vi "NotifyIcon - Example 2.vi"() -> ()   [LabVIEW 2018]
uses:
  TypeDefs/NotifyIcon Events.ctl
  TypeDefs/NotifyIcon Event Registration Actions.ctl
  System.Windows.Forms
panel:
  in  "Events to register":T1[](array[typedef])=[enum."BalloonTipClosed"]
  in  "Add to Event Registration":bool
  in  "Checked":bool
  in  "Visible":bool=TRUE
  in  "Context MenuItem":string="submenu\\subitem1"
  in  "Change MenuItem Properties":bool
  in  "New Icon File Path":path=path "C:/Program Files/National Instruments/LabVIEW 2009/applibs/lvapp.ico"
  in  "Change Icon":bool
  in  "Context Menu":string[][](array[string])=[["<submenu2>", "<submenu1>", "<submenu2>"], ["<submenu1>", "subitem1", "subitem1"], ["item1", "subitem2", "subitem2"], ["item2", "", "subitem3"], ["-", "", ""], ["Exit", "", ""]]
  in  "Change Context Menu":bool
  in  "Text":string="Baloon Tip Text"
  in  "Title":string="Balloon Tip"
  in  "Icon (None)":i32(ring)=1 items=["None", "Info", "Warning", "Error"]
  in  "Show Balloon Tip":bool
  in  "stop":bool
  in  "Icon File Path (set to valid path before running)":path=path "C:/Program Files/National Instruments/LabVIEW 2009/applibs/lvapp.ico"
  # "**Warning - if you register a new event, you need to handle the\nevent in the Case Structure found in the NotifyIcon User Event.\n\nIf you do not, you will recieve error 7000"
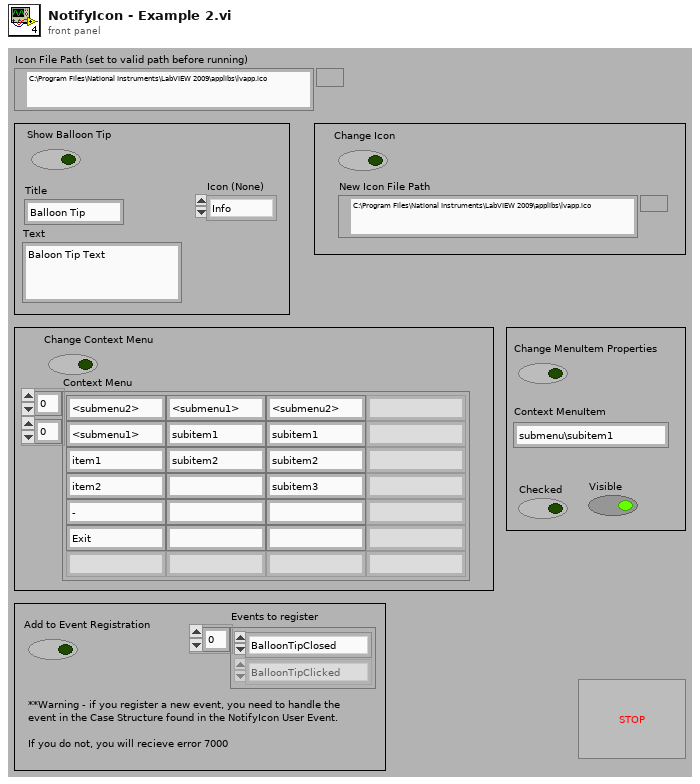
[diagram p1: front panel]
types:
  T1 = typedef "NotifyIcon Events.ctl" = enum16{"BalloonTipClicked", "BalloonTipClosed", "BalloonTipShown", "Click", "Disposed", "DoubleClick", "MouseClick", "MouseDoubleClick", "MouseDown", "MouseMove", "MouseUp", "MenuItemClick", "MenuItemSelect"}
  T2 = typedef "NotifyIcon Event Registration Actions.ctl" = enum16{"Initial Event Registration", "Add to Event Registration", "Destroy Events and Re-register"}
  T3 = typedef "NotifyIcon Event Data.ctl" = cluster{"NotifyIcon Event":T1, "Data String":string}
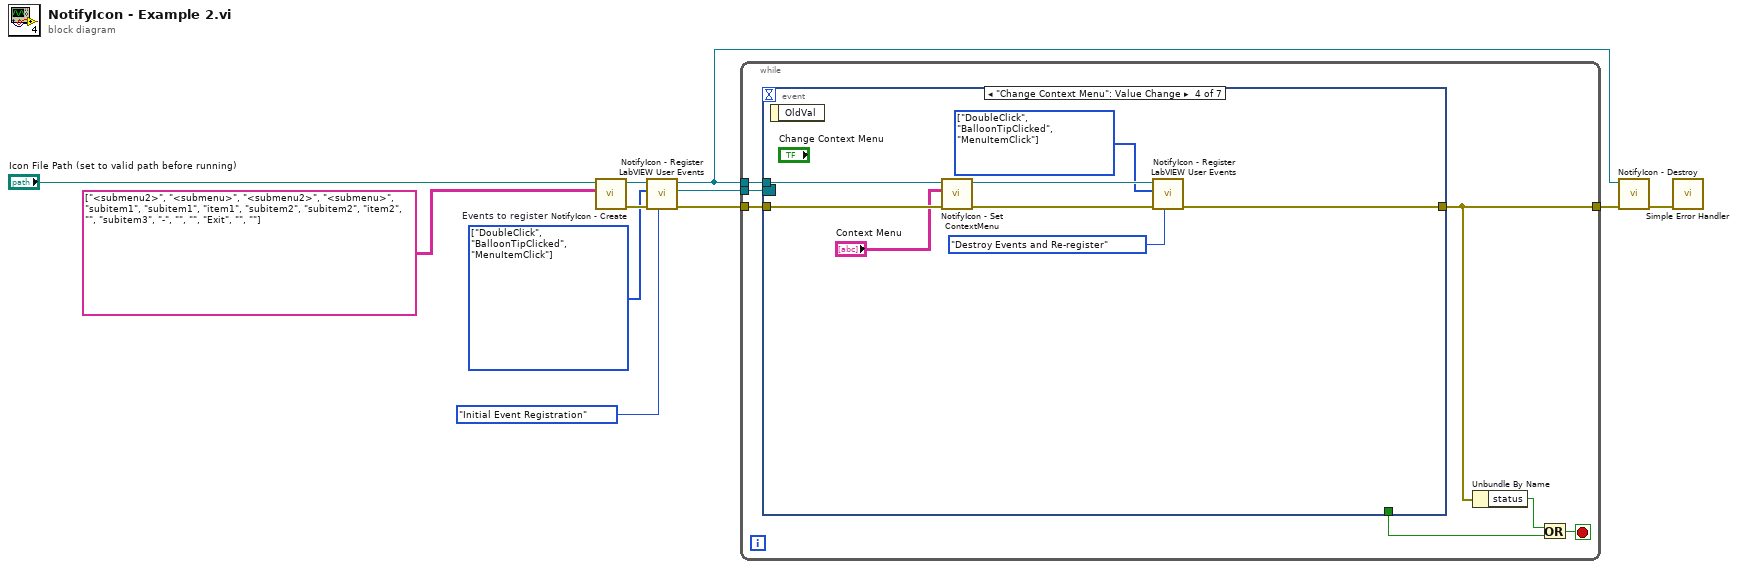
[diagram p0: block diagram]
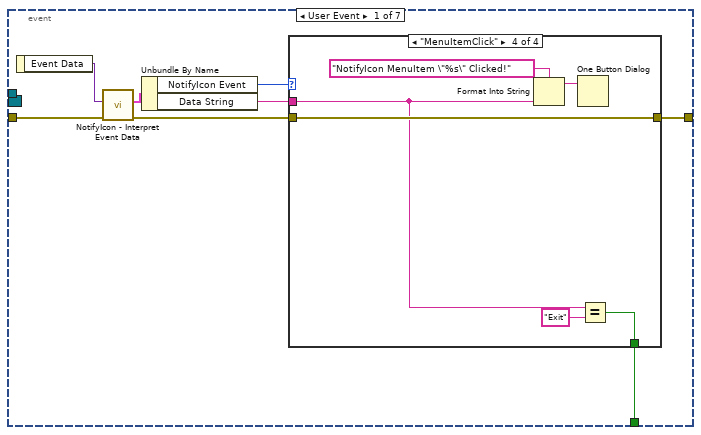
[diagram p2: hidden frame]
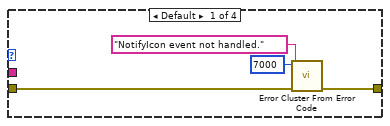
[diagram p3: hidden frame]
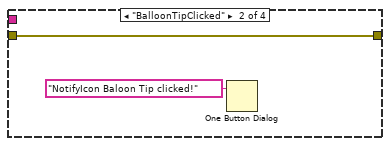
[diagram p4: hidden frame]
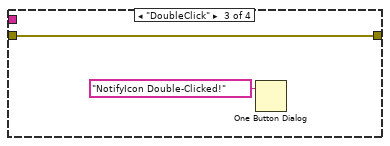
[diagram p5: hidden frame]
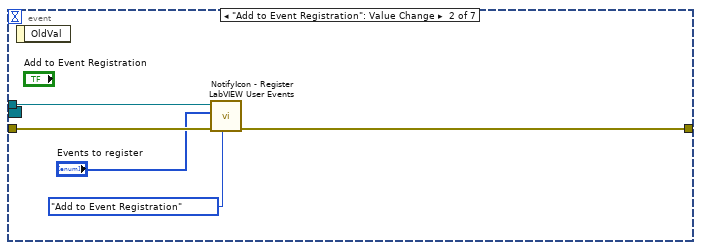
[diagram p6: hidden frame]
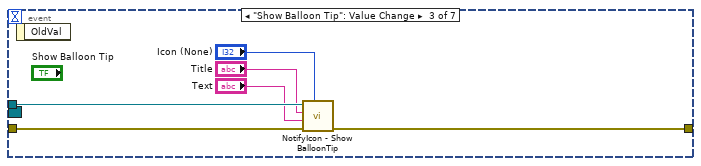
[diagram p7: hidden frame]
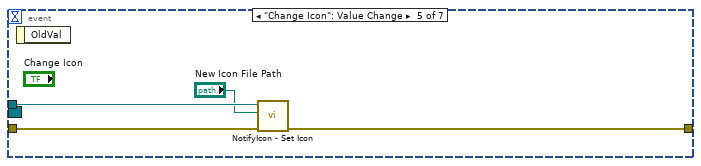
[diagram p8: hidden frame]
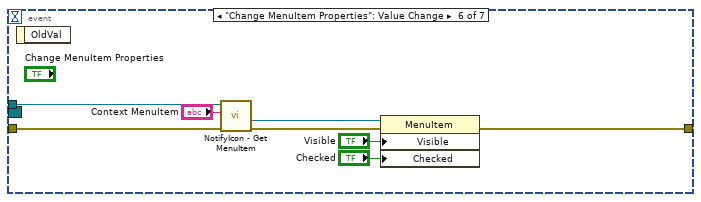
[diagram p9: hidden frame]
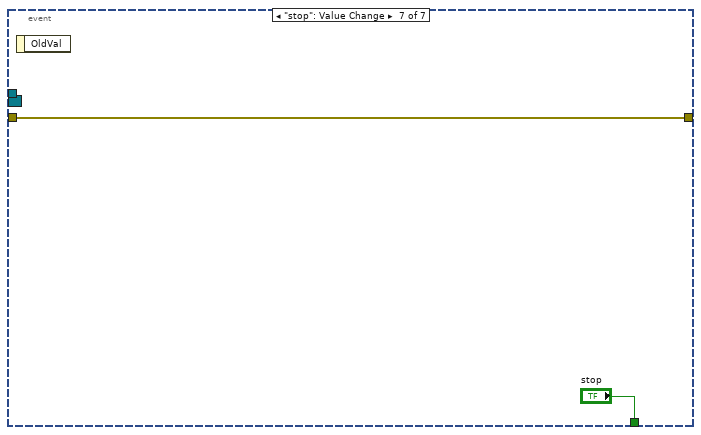
[diagram p10: hidden frame]
diagram:
  w8 = T1[] [enum."DoubleClick", enum."BalloonTipClicked", enum."MenuItemClick"] items=["BalloonTipClicked", "BalloonTipClosed", "BalloonTipShown", "Click", "Disposed", "DoubleClick", "MouseClick", "MouseDoubleClick", "MouseDown", "MouseMove", "MouseUp", "MenuItemClick", "MenuItemSelect"]  # Events to register
  n1 = call "NotifyIcon - Create.vi"("Context Menu (optional)"=string[][] [["<submenu2>", "<submenu>", "<submenu2>"], ["<submenu>", "subitem1", "subitem1"], ["item1", "subitem2", "subitem2"], ["item2", "", "subitem3"], ["-", "", ""], ["Exit", "", ""]], "Icon File Path"="Icon File Path (set to valid path before running)") -> ("error out"=w9:errorcluster, "NotifyIcon reference"=w11:refnum<k24>)  [unwired: 8 in]
  n2 = call "NotifyIcon - Register LabVIEW User Events.vi"("Action"=NotifyIcon_Event_Registration_Actions."Initial Event Registration", "error in"=w9, "Events to register"=w8, "NotifyIcon reference in"=w11) -> ("error out"=w5:errorcluster, "Event Registration Refnum"=w6:refnum<event-registration>, "NotifyIcon reference out"=w2:refnum<k24>)  [unwired: 5 in]
  n3 = while {
    tunnel: w6 -> [w18]
    tunnel: w2 -> [w17]
    tunnel: w5 -> [w16]
    tunnel: [w12] -> w4
    stop <- w13 stop-if-true
    n4 = event shown="[3] \"Change Context Menu\": Value Change" {
      selector: w18 -> [_ _ _ _ _ _ _]
      dyn-events: _ -> [_ _ _ _ _ _ _]
      timeout: _ -> [_ _ _ _ _ _ _]
      tunnel: w17 -> [_ w45 w50 w58 w63 w70 _]
      tunnel: w16 -> [w26 w44 w51 w59 w62 w71 w72]
      tunnel: [w19 _ _ _ _ _ "stop"] -> w15
      tunnel: [w21 w42 w46 w52 w60 w67 w72] -> w12
      event User Event {
        n5 = event-data() -> ("Event Data"=w25:variant)  [unwired: 1 in]
        n6 = call "NotifyIcon - Interpret Event Data.vi"("error in"=w26, "NotifyIcon Event Data"=w25) -> ("error out"=w22:errorcluster, "NotifyIcon Event Data"=w24:T3)  [unwired: 8 in]
        n7 = Unbundle By Name(w24) -> ("NotifyIcon Event"=w23:T1, "Data String"=w20:string)
        n8 = case shown="\"MenuItemClick\"" w23 {
          tunnel: w22 -> [w29 w31 w34 w39]
          tunnel: [w30 w31 w34 w39] -> w21
          tunnel: w20 -> [_ _ _ w37]
          tunnel: [_ _ _ w35] -> w19
          frame Default {
            n9 = call <vilib>:"Error Cluster From Error Code.vi"("error in (no error)"=w29, "error message (\"\")"="NotifyIcon event not handled." ("error message (\"\")"), "error code (0)"=7000) -> ("error out"=w30:errorcluster)  [unwired: 6 in]
          }
          frame "BalloonTipClicked" {
            n10 = One Button Dialog(message="NotifyIcon Baloon Tip clicked!") -> ()  [unwired: 1 in, 1 out]
          }
          frame "DoubleClick" {
            n11 = One Button Dialog(message="NotifyIcon Double-Clicked!") -> ()  [unwired: 1 in, 1 out]
          }
          frame "MenuItemClick" {
            n12 = Format Into String(format string="NotifyIcon MenuItem \"%s\" Clicked!", w37) -> (resulting string=w38:string)  [unwired: 2 in, 1 out]
            n13 = One Button Dialog(message=w38) -> ()  [unwired: 1 in, 1 out]
            n14 = Equal?(x=w37, y="Exit") -> (x = y?=w35:bool)
          }
        }
      }
      event "Add to Event Registration": Value Change {
        n15 = event-data() -> ()  [unwired: 1 in, 1 out]
        n16 = call "NotifyIcon - Register LabVIEW User Events.vi"("Action"=NotifyIcon_Event_Registration_Actions."Add to Event Registration", "error in"=w44, "Events to register"="Events to register", "NotifyIcon reference in"=w45) -> ("error out"=w42:errorcluster)  [unwired: 5 in, 2 out]
      }
      event "Show Balloon Tip": Value Change {
        n17 = event-data() -> ()  [unwired: 1 in, 1 out]
        n18 = call "NotifyIcon - Show BalloonTip.vi"("Icon (None)"="Icon (None)", "error in"=w51, "Text"="Text", "Title"="Title", "NotifyIcon reference in"=w50) -> ("error out"=w46:errorcluster)  [unwired: 5 in, 1 out]
      }
      event "Change Context Menu": Value Change {
        w53 = T1[] [enum."DoubleClick", enum."BalloonTipClicked", enum."MenuItemClick"] items=["BalloonTipClicked", "BalloonTipClosed", "BalloonTipShown", "Click", "Disposed", "DoubleClick", "MouseClick", "MouseDoubleClick", "MouseDown", "MouseMove", "MouseUp", "MenuItemClick", "MenuItemSelect"] ("Events to register")
        n19 = event-data() -> ()  [unwired: 1 in, 1 out]
        n20 = call "NotifyIcon - Set ContextMenu.vi"("error in"=w59, "Context Menu"="Context Menu", "NotifyIcon reference in"=w58) -> ("error out"=w55:errorcluster, "NotifyIcon reference out"=w56:refnum<k24>)  [unwired: 7 in]
        n21 = call "NotifyIcon - Register LabVIEW User Events.vi"("Action"=NotifyIcon_Event_Registration_Actions."Destroy Events and Re-register", "error in"=w55, "Events to register"=w53, "NotifyIcon reference in"=w56) -> ("error out"=w52:errorcluster)  [unwired: 5 in, 2 out]
      }
      event "Change Icon": Value Change {
        n22 = event-data() -> ()  [unwired: 1 in, 1 out]
        n23 = call "NotifyIcon - Set Icon.vi"("error in"=w62, "Icon File Path"="New Icon File Path", "NotifyIcon reference in"=w63) -> ("error out"=w60:errorcluster)  [unwired: 7 in, 1 out]
      }
      event "Change MenuItem Properties": Value Change {
        n24 = event-data() -> ()  [unwired: 1 in, 1 out]
        n25 = call "NotifyIcon - Get MenuItem.vi"("error in"=w71, "Context MenuItem"="Context MenuItem", "NotifyIcon reference in"=w70) -> ("error out"=w68:errorcluster, "MenuItem reference"=w64:refnum<k24>)  [unwired: 6 in, 1 out]
        n26 = property class="MenuItem"(reference=w64, error in=w68, "Visible"="Visible", "Checked"="Checked") -> (error out=w67:errorcluster)  [unwired: 1 out]
      }
      event "stop": Value Change {
        n27 = event-data() -> ()  [unwired: 1 in, 1 out]
      }
    }
    n28 = Unbundle By Name(w12) -> ("status"=w14:bool)
    n29 = Or(x=w14, y=w15) -> (x .or. y?=w13:bool)
  }
  n30 = call "NotifyIcon - Destroy.vi"("error in"=w4, "NotifyIcon reference"=w2) -> ("error out"=w3:errorcluster)  [unwired: 9 in]
  n31 = call <vilib>:"Simple Error Handler.vi"("error in (no error)"=w3) -> ()  [unwired: 4 in, 5 out]
